vi "REPORT TXT.vi"(6 "Dati collaudo":T1, 8 "template (empty)":path, 9 "BOLLETTINO":string[][](array[string]), 10 "Codice":string, 11 "report file path":path) -> ()   [LabVIEW 2019]
uses:
  <vilib>/Utility/NIReport.llb/NI_report.lvclass
  <vilib>/addons/_office/NI_ReportGenerationToolkit.lvlib
  <vilib>/Utility/NIReport.llb/Excel/NI_Excel.lvclass
  <vilib>/addons/database/NI_Database_API.lvlib
  <vilib>/addons/database/_DB Variant To Data/Database Variant To Data.xnode
  Global percorso impostazioni.vi
  <vilib>/addons/_office/excel.llb/Excel Easy Table (str).vi
  <vilib>/Utility/file.llb/Write Delimited Spreadsheet (string).vi
  TypeDef/Dati collaudo.ctl
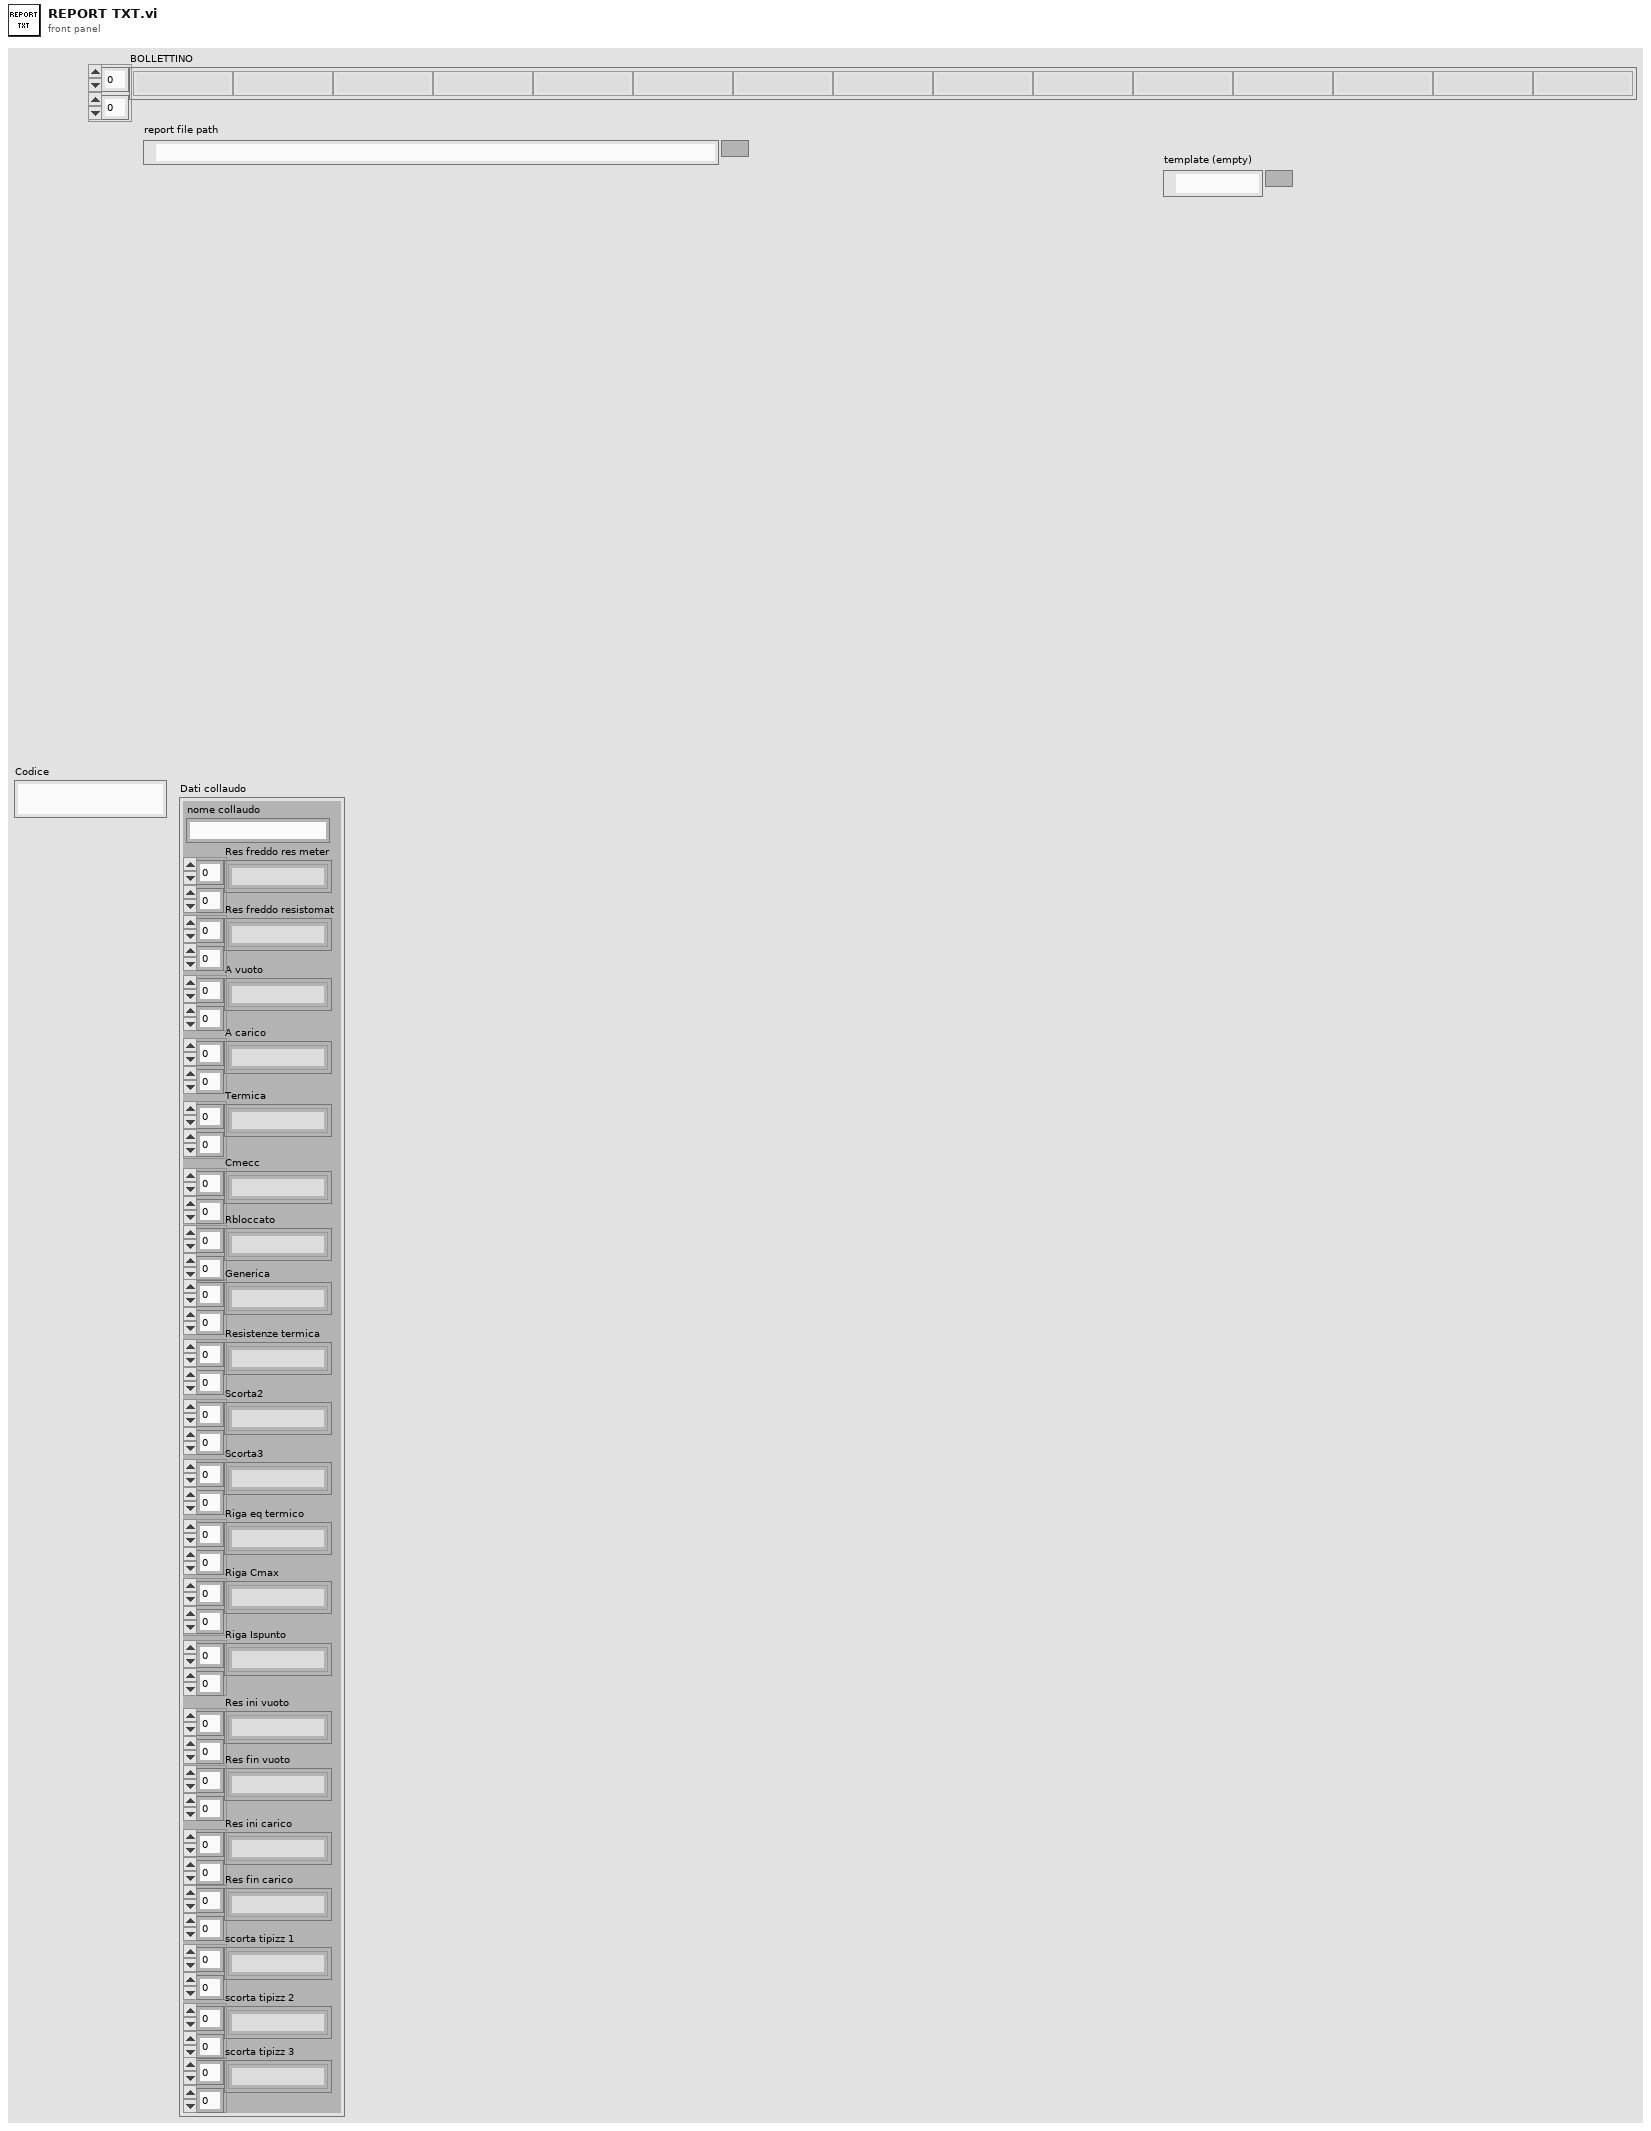
[diagram p1: front panel]
types:
  T1 = typedef "Dati collaudo.ctl" = cluster{"nome collaudo":string, "Res freddo res meter":string[][], "Res freddo resistomat":string[][], "A vuoto":string[][], "A carico":string[][], "Termica":string[][], "Cmecc":string[][], "Rbloccato":string[][], "Generica":string[][], "Resistenze termica":string[][], "Scorta2":string[][], "Scorta3":string[][], "Riga eq termico":string[][], "Riga Cmax":string[][], "Riga Ispunto":string[][], "Res ini vuoto":string[][], "Res fin vuoto":string[][], "Res ini carico":string[][], "Res fin carico":string[][], "scorta tipizz 1":string[][], "scorta tipizz 2":string[][], "scorta tipizz 3":string[][]}
  T2 = cluster{"BANCO":string, "ANNO":string, "PROGRESSIVO":string, "TIPO PROVA":string, "PROVA SPECIALE ?":string, "DATA":string}
  T3 = typedef "NI_Database_API.lvlib/Conn ObjectReference.ctl" = refnum<k1>
  T4 = typedef "Curve prova.ctl" = cluster{"Curva 1":string[][], "Curva 2":string[][], "Curva 3":string[][]}
  T5 = enum16{"maximized", "minimized", "normal", "no change"}
  T6 = enum16{"Standard Report", "HTML", "Word", "Excel"}
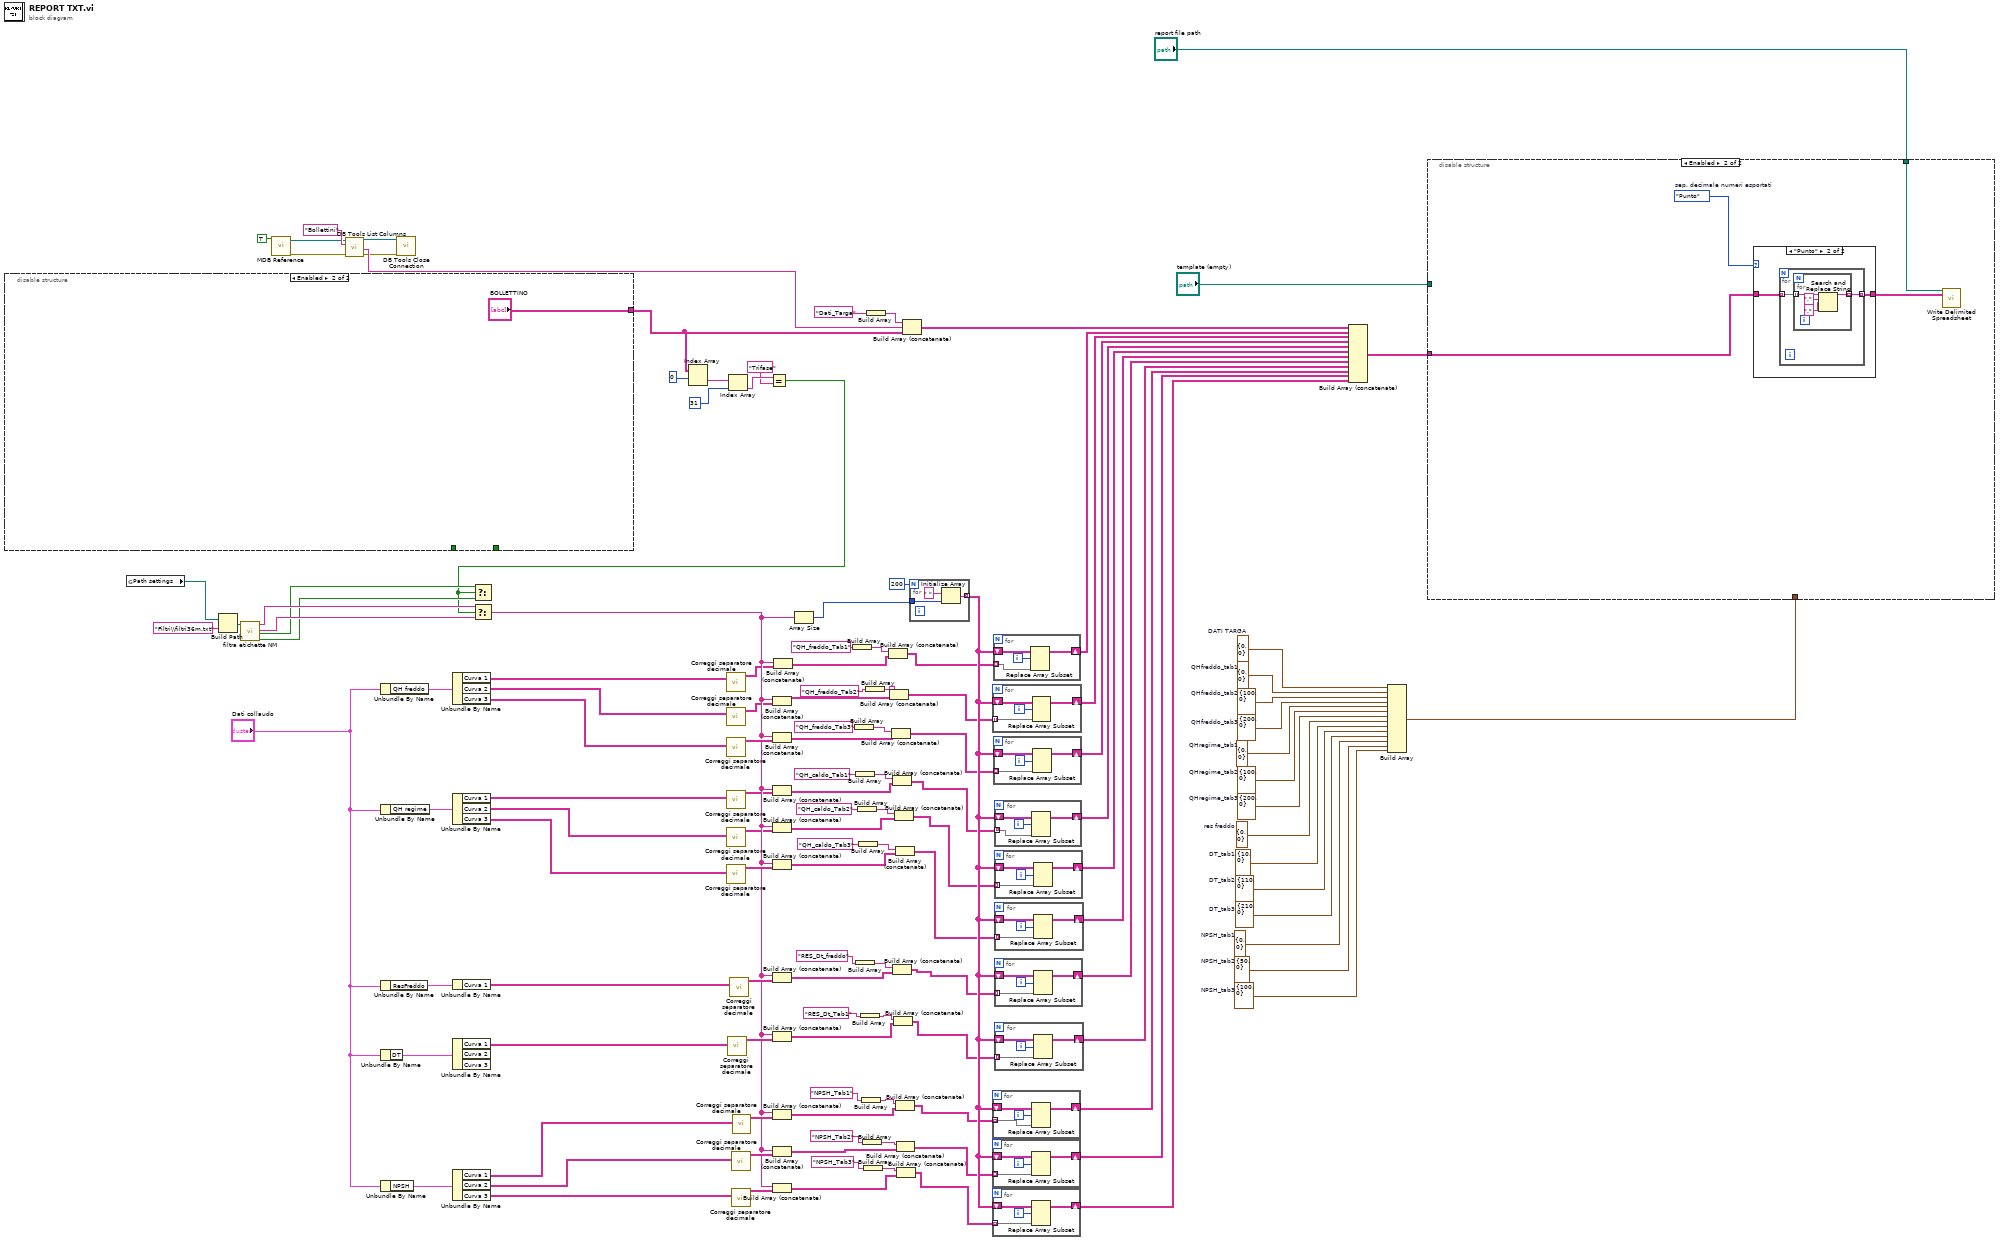
[diagram p0: block diagram]
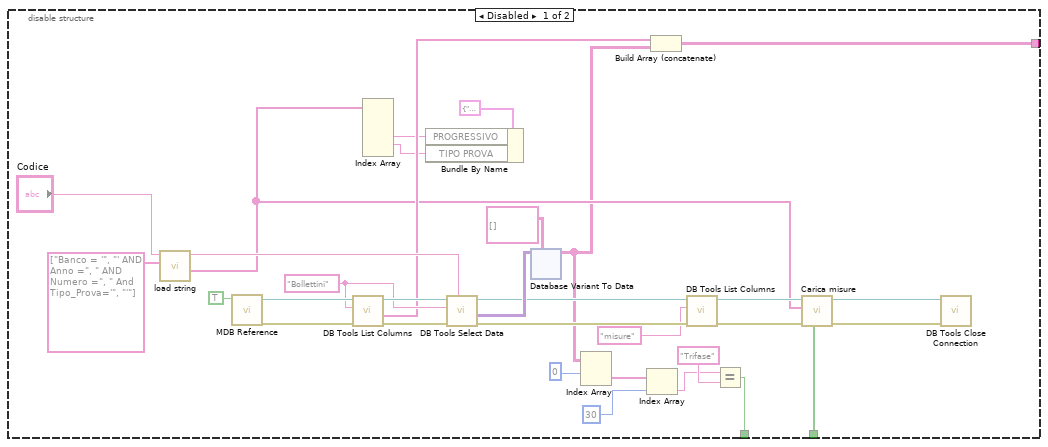
[diagram p2: hidden frame]
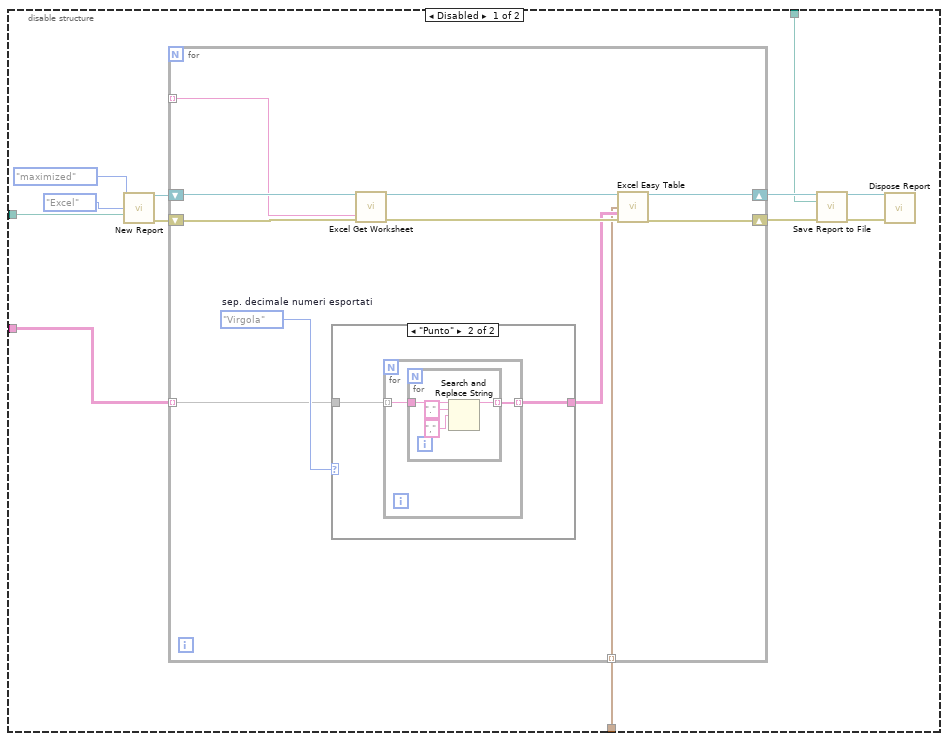
[diagram p3: hidden frame]
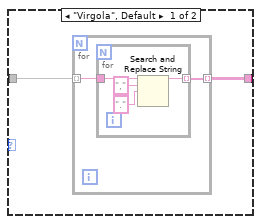
[diagram p4: hidden frame]
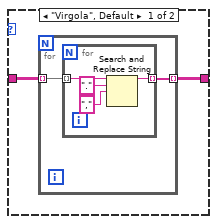
[diagram p5: hidden frame]
diagram:
  w114 = cluster{"row":i32, "column":i32} {"row"=100, "column"=0}  # NPSH_tab3
  w115 = cluster{"row":i32, "column":i32} {"row"=50, "column"=0}  # NPSH_tab2
  w116 = cluster{"row":i32, "column":i32} {"row"=0, "column"=0}  # NPSH_tab1
  w117 = cluster{"row":i32, "column":i32} {"row"=210, "column"=0}  # DT_tab3
  w118 = cluster{"row":i32, "column":i32} {"row"=110, "column"=0}  # DT_tab2
  w119 = cluster{"row":i32, "column":i32} {"row"=10, "column"=0}  # DT_tab1
  w120 = cluster{"row":i32, "column":i32} {"row"=0, "column"=0}  # res freddo
  w121 = cluster{"row":i32, "column":i32} {"row"=200, "column"=0}  # QHregime_tab3
  w122 = cluster{"row":i32, "column":i32} {"row"=100, "column"=0}  # QHregime_tab2
  w123 = cluster{"row":i32, "column":i32} {"row"=0, "column"=0}  # QHregime_tab1
  w124 = cluster{"row":i32, "column":i32} {"row"=200, "column"=0}  # QHfreddo_tab3
  w125 = cluster{"row":i32, "column":i32} {"row"=100, "column"=0}  # QHfreddo_tab2
  w126 = cluster{"row":i32, "column":i32} {"row"=0, "column"=0}  # QHfreddo_tab1
  w127 = cluster{"row":i32, "column":i32} {"row"=0, "column"=0}  # DATI TARGA
  n1 = disable-structure shown="Enabled" {
    disable-tunnel: [w132 _] -> _
    disable-tunnel: _ -> [w131 _]
    disable-tunnel: [w130 "BOLLETTINO"] -> w20
    frame Disabled {
      w152 = "Bollettini" ("table")
      n2 = call "load string.vi"("Array in"=string[] ["Banco = '", "' AND Anno =", " AND Numero =", " And Tipo_Prova='", "'"], "Codice"="Codice") -> ("ID bollettino"=w139:string[], "String command"=w157:string)  [unwired: 7 in, 1 out]
      n3 = call "MDB Reference.vi"("Collaudi T/motori F"=TRUE ("NM?")) -> ("error out"=w154:errorcluster, "Refnum out"=w156:T3)  [unwired: 8 in, 1 out]
      n4 = call <vilib>:"DB Tools List Columns.vi"("error in (no error)"=w154, "table"=w152, "connection reference"=w156) -> ("error out"=w153:errorcluster, "columns"=w151:string[], "connection reference out"=w155:T3)  [unwired: 1 in, 1 out]
      n5 = Index Array(array=w139) -> (element #3=w146:string, element #4=w145:string)  [unwired: 5 in, 3 out]
      n6 = Bundle By Name(cluster=T2 {"BANCO"="0", "ANNO"="17", "PROGRESSIVO"="12", "TIPO PROVA"="F", "PROVA SPECIALE ?"="NO", "DATA"="29/11/2017 10:25:21"} ("bollettino"), "PROGRESSIVO"=w146, "TIPO PROVA"=w145) -> ()  [unwired: 1 out]
      n7 = call <vilib>:"DB Tools Select Data.vi"("condition"=w157, "error in (no error)"=w153, "table"=w152, "connection reference"=w155) -> ("error out"=w150:errorcluster, "data"=w159:variant[][], "connection reference out"=w149:T3)  [unwired: 2 in]
      n8 = xnode "Database Variant To Data"("database variant"=w159, "type"=string[][] [] ("Item Names")) -> ("data"=w133:string[][])  [unwired: 1 in, 1 out]
      n9 = Index Array(array=w133, index (row)=0 ("disabled index (col)")) -> (element=w135:string[])  [unwired: 1 in]
      n10 = Index Array(array=w135, index=30) -> (element=w137:string)
      n11 = Build Array (concatenate)(w151, w133) -> (w130:string[][])
      n12 = call <vilib>:"DB Tools List Columns.vi"("error in (no error)"=w150, "table"="misure", "connection reference"=w149) -> ("error out"=w144:errorcluster, "connection reference out"=w143:T3)  [unwired: 1 in, 2 out]
      n13 = Equal?(x=w137, y="Trifase") -> (x = y?=w132:bool)
      n14 = call "Carica misure.vi"("Filtro 3ph6ch"=w131, "error in (no error)"=w144, "ID bollettino"=w139, "Refnum in"=w143) -> ("error out"=w141:errorcluster, "Refnum out"=w142:T3)  [unwired: 5 in, 1 out]
      n15 = call <vilib>:"DB Tools Close Connection.vi"("error in (no error)"=w141, "connection reference"=w142) -> ()  [unwired: 5 in, 1 out]
    }
    frame Enabled {
    }
  }
  n16 = global read "Global percorso impostazioni.vi" "Path settings"() -> (w1:path)
  n17 = Build Path(base path=w1, name or relative path="Filtri\\filtri36m.txt") -> (appended path=w110:path)
  n18 = call "filtra etichette NM.vi"("File filtri path"=w110) -> ("Array 3ph3ch"=w109:string[], "Array 1ph"=w108:string[], "Filtro 3ph3ch"=w107:bool[], "Filtro 1ph"=w106:bool[])  [unwired: 11 in, 4 out]
  n19 = call "MDB Reference.vi"("Collaudi T/motori F"=TRUE ("NM?")) -> ("error out"=w32:errorcluster, "Refnum out"=w31:T3)  [unwired: 8 in, 1 out]
  n20 = call <vilib>:"DB Tools List Columns.vi"("error in (no error)"=w32, "table"="Bollettini", "connection reference"=w31) -> ("error out"=w27:errorcluster, "columns"=w28:string[], "connection reference out"=w26:T3)  [unwired: 1 in, 1 out]
  n21 = Unbundle By Name("Dati collaudo") -> ("QH freddo"=w101:T4)
  n22 = Unbundle By Name("Dati collaudo") -> ("QH regime"=w102:T4)
  n23 = Unbundle By Name("Dati collaudo") -> ("ResFreddo"=w104:cluster{"Curva 1":string[][]})
  n24 = Unbundle By Name("Dati collaudo") -> ("DT"=w103:T4)
  n25 = Unbundle By Name("Dati collaudo") -> ("NPSH"=w105:T4)
  n26 = call <vilib>:"DB Tools Close Connection.vi"("error in (no error)"=w27, "connection reference"=w26) -> ()  [unwired: 5 in, 1 out]
  n27 = Unbundle By Name(w101) -> ("Curva 1"=w10:string[][], "Curva 2"=w8:string[][], "Curva 3"=w16:string[][])
  n28 = Unbundle By Name(w102) -> ("Curva 1"=w12:string[][], "Curva 2"=w14:string[][], "Curva 3"=w15:string[][])
  n29 = Unbundle By Name(w104) -> ("Curva 1"=w6:string[][])
  n30 = Unbundle By Name(w103) -> ("Curva 1"=w5:string[][])  [unwired: 2 out]
  n31 = Unbundle By Name(w105) -> ("Curva 1"=w4:string[][], "Curva 2"=w3:string[][], "Curva 3"=w2:string[][])
  n32 = Index Array(array=w20, index (row)=0 ("disabled index (col)")) -> (element=w24:string[])  [unwired: 1 in]
  n33 = call "Correggi separatore decimale.vi"("Array in"=w10) -> ("Array out"=w9:string[][])  [unwired: 10 in]
  n34 = call "Correggi separatore decimale.vi"("Array in"=w8) -> ("Array out"=w7:string[][])  [unwired: 10 in]
  n35 = call "Correggi separatore decimale.vi"("Array in"=w16) -> ("Array out"=w99:string[][])  [unwired: 10 in]
  n36 = call "Correggi separatore decimale.vi"("Array in"=w12) -> ("Array out"=w11:string[][])  [unwired: 10 in]
  n37 = call "Correggi separatore decimale.vi"("Array in"=w14) -> ("Array out"=w13:string[][])  [unwired: 10 in]
  n38 = call "Correggi separatore decimale.vi"("Array in"=w15) -> ("Array out"=w98:string[][])  [unwired: 10 in]
  n39 = call "Correggi separatore decimale.vi"("Array in"=w5) -> ("Array out"=w96:string[][])  [unwired: 10 in]
  n40 = Index Array(array=w24, index=31) -> (element=w22:string)
  n41 = call "Correggi separatore decimale.vi"("Array in"=w6) -> ("Array out"=w97:string[][])  [unwired: 10 in]
  n42 = call "Correggi separatore decimale.vi"("Array in"=w3) -> ("Array out"=w94:string[][])  [unwired: 10 in]
  n43 = call "Correggi separatore decimale.vi"("Array in"=w2) -> ("Array out"=w95:string[][])  [unwired: 10 in]
  n44 = call "Correggi separatore decimale.vi"("Array in"=w4) -> ("Array out"=w93:string[][])  [unwired: 10 in]
  n45 = Equal?(x=w22, y="Trifase") -> (x = y?=w19:bool)
  n46 = Select(t=w107, s=w19, f=w106) -> ()  [unwired: 1 out]
  n47 = Select(t=w109, s=w19, f=w108) -> (s? t:f=w17:string[])
  n48 = Build Array (concatenate)(w17, w7) -> (w73:string[][])
  n49 = Build Array (concatenate)(w17, w99) -> (w67:string[][])
  n50 = Build Array (concatenate)(w17, w11) -> (w64:string[][])
  n51 = Build Array (concatenate)(w17, w13) -> (w57:string[][])
  n52 = Build Array (concatenate)(w17, w98) -> (w55:string[][])
  n53 = Build Array (concatenate)(w17, w97) -> (w52:string[][])
  n54 = Build Array (concatenate)(w17, w96) -> (w49:string[][])
  n55 = Build Array (concatenate)(w17, w93) -> (w44:string[][])
  n56 = Build Array (concatenate)(w17, w94) -> (w39:string[][])
  n57 = Build Array (concatenate)(w17, w95) -> (w35:string[][])
  n58 = Build Array (concatenate)(w17, w9) -> (w75:string[][])
  n59 = Array Size(array=w17) -> (size(s)=w18:i32)
  n60 = Build Array("QH_freddo_Tab1") -> (w77:string[])
  n61 = Build Array("QH_freddo_Tab3") -> (w68:string[])
  n62 = Build Array("QH_caldo_Tab1") -> (w65:string[])
  n63 = Build Array("RES_Dt_freddo") -> (w53:string[])
  n64 = Build Array("QH_caldo_Tab2") -> (w60:string[])
  n65 = Build Array("QH_caldo_Tab3") -> (w59:string[])
  n66 = Build Array("RES_Dt_Tab1") -> (w46:string[])
  n67 = Build Array("NPSH_Tab1") -> (w45:string[])
  n68 = Build Array("NPSH_Tab2") -> (w40:string[])
  n69 = Build Array("NPSH_Tab3") -> (w37:string[])
  n70 = Build Array("QH_freddo_Tab2") -> (w71:string[])
  n71 = Build Array("Dati_Targa") -> (w29:string[])
  n72 = Build Array (concatenate)(w77, w75) -> (w74:string[][])
  n73 = Build Array (concatenate)(w71, w73) -> (w72:string[][])
  n74 = Build Array (concatenate)(w68, w67) -> (w66:string[][])
  n75 = Build Array (concatenate)(w65, w64) -> (w63:string[][])
  n76 = Build Array (concatenate)(w53, w52) -> (w51:string[][])
  n77 = Build Array (concatenate)(w46, w49) -> (w48:string[][])
  n78 = Build Array (concatenate)(w60, w57) -> (w56:string[][])
  n79 = Build Array (concatenate)(w59, w55) -> (w54:string[][])
  n80 = Build Array (concatenate)(w45, w44) -> (w43:string[][])
  n81 = Build Array (concatenate)(w40, w39) -> (w38:string[][])
  n82 = Build Array (concatenate)(w37, w35) -> (w34:string[][])
  n83 = Build Array (concatenate)(w29, w28, w20) -> (w82:string[][])
  n84 = for {
    N: 200 -> [_]
    tunnel: w18 -> [w208]
    tunnel: [w207] -> w80 mode=indexing
    n85 = Initialize Array(" ", w208) -> (w207:string[])
  }
  n86 = for {
    shift-right: [w211] -> w85
    shift-left: w80 -> [w213]
    tunnel: w43 -> [w210] mode=indexing
    i -> [w212]
    n87 = Replace Array Subset(array=w213, new element=w210, index (row)=w212) -> (w211:string[][])  [unwired: 1 in]
  }
  n88 = for {
    shift-right: [w215] -> w84
    shift-left: w80 -> [w217]
    tunnel: w38 -> [w214] mode=indexing
    i -> [w216]
    n89 = Replace Array Subset(array=w217, new element=w214, index (row)=w216) -> (w215:string[][])  [unwired: 1 in]
  }
  n90 = for {
    shift-right: [w219] -> w83
    shift-left: w80 -> [w221]
    tunnel: w34 -> [w218] mode=indexing
    i -> [w220]
    n91 = Replace Array Subset(array=w221, new element=w218, index (row)=w220) -> (w219:string[][])  [unwired: 1 in]
  }
  n92 = for {
    shift-right: [w223] -> w90
    shift-left: w80 -> [w225]
    tunnel: w72 -> [w222] mode=indexing
    i -> [w224]
    n93 = Replace Array Subset(array=w225, new element=w222, index (row)=w224) -> (w223:string[][])  [unwired: 1 in]
  }
  n94 = for {
    tunnel: w74 -> [w228] mode=indexing
    shift-right: [w226] -> w91
    shift-left: w80 -> [w229]
    i -> [w227]
    n95 = Replace Array Subset(array=w229, new element=w228, index (row)=w227) -> (w226:string[][])  [unwired: 1 in]
  }
  n96 = for {
    shift-right: [w231] -> w89
    shift-left: w80 -> [w233]
    tunnel: w66 -> [w230] mode=indexing
    i -> [w232]
    n97 = Replace Array Subset(array=w233, new element=w230, index (row)=w232) -> (w231:string[][])  [unwired: 1 in]
  }
  n98 = for {
    shift-right: [w235] -> w87
    shift-left: w80 -> [w237]
    tunnel: w56 -> [w234] mode=indexing
    i -> [w236]
    n99 = Replace Array Subset(array=w237, new element=w234, index (row)=w236) -> (w235:string[][])  [unwired: 1 in]
  }
  n100 = for {
    shift-right: [w239] -> w78
    shift-left: w80 -> [w241]
    tunnel: w51 -> [w238] mode=indexing
    i -> [w240]
    n101 = Replace Array Subset(array=w241, new element=w238, index (row)=w240) -> (w239:string[][])  [unwired: 1 in]
  }
  n102 = for {
    tunnel: w63 -> [w244] mode=indexing
    shift-right: [w242] -> w88
    shift-left: w80 -> [w245]
    i -> [w243]
    n103 = Replace Array Subset(array=w245, new element=w244, index (row)=w243) -> (w242:string[][])  [unwired: 1 in]
  }
  n104 = for {
    shift-right: [w247] -> w86
    shift-left: w80 -> [w249]
    tunnel: w54 -> [w246] mode=indexing
    i -> [w248]
    n105 = Replace Array Subset(array=w249, new element=w246, index (row)=w248) -> (w247:string[][])  [unwired: 1 in]
  }
  n106 = for {
    shift-right: [w251] -> w79
    shift-left: w80 -> [w253]
    tunnel: w48 -> [w250] mode=indexing
    i -> [w252]
    n107 = Replace Array Subset(array=w253, new element=w250, index (row)=w252) -> (w251:string[][])  [unwired: 1 in]
  }
  n108 = Build Array (concatenate)(w82, w91, w90, w89, w88, w87, w86, w78, w79, w85, w84, w83) -> (w128:string[][])
  n109 = Build Array(w127, w126, w125, w124, w123, w122, w121, w120, w119, w118, w117, w116, w115, w114) -> (w113:cluster{"row":i32, "column":i32}[])
  n110 = disable-structure shown="Enabled" {
    disable-tunnel: "template (empty)" -> [w266 _]
    disable-tunnel: w128 -> [w261 w294]
    disable-tunnel: w113 -> [w259 _]
    disable-tunnel: "report file path" -> [w254 w297]
    frame Disabled {
      n111 = call <vilib>:"New Report.vi"("window state (normal)"=T5."maximized", "report type"=T6."Excel", "template (empty)"=w266) -> ("report out"=w264:refnum<class "NI_report.lvclass">, "error out"=w262:errorcluster)  [unwired: 11 in]
      n112 = for {
        shift-right: [w277] -> w256
        shift-left: w264 -> [w276]
        tunnel: [w274] -> w263 mode=indexing
        shift-right: [w271] -> w258
        shift-left: w262 -> [w273]
        tunnel: w261 -> [w269] mode=indexing
        tunnel: w259 -> [w267] mode=indexing
        w270 = enum16{"Virgola", "Punto"}."Virgola"  # sep. decimale numeri esportati
        n113 = case shown="\"Punto\"" w270 {
          tunnel: w269 -> [w279 w287]
          tunnel: [w278 w286] -> w268
          frame "Virgola", Default {
            n114 = for {
              tunnel: w279 -> [w281] mode=indexing
              tunnel: [w280] -> w278 mode=indexing
              n115 = for {
                tunnel: w281 -> [w285]
                tunnel: [w282] -> w280 mode=indexing
                n116 = Search and Replace String(input string=w285, search string=",", replace string="." ("search string")) -> (result string=w282:string)  [unwired: 5 in, 3 out]
              }
            }
          }
          frame "Punto" {
            n117 = for {
              tunnel: w287 -> [w289] mode=indexing
              tunnel: [w288] -> w286 mode=indexing
              n118 = for {
                tunnel: w289 -> [w293]
                tunnel: [w290] -> w288 mode=indexing
                n119 = Search and Replace String(input string=w293, search string=".", replace string="," ("search string")) -> (result string=w290:string)  [unwired: 5 in, 3 out]
              }
            }
          }
        }
        n120 = call <vilib>:"Excel Get Worksheet.vi"("report in"=w276, "error in (no error)"=w273, "name (\"\")"=w274) -> ("report out"=w275:refnum<class "NI_report.lvclass">, "error out"=w272:errorcluster)  [unwired: 11 in]
        n121 = call-poly <vilib>:"Excel Easy Table.vi"("report in"=w275, "start (0, 0)"=w267, "text data"=w268, "error in (no error)"=w272) -> ("report out"=w277:refnum<class "NI_report.lvclass">, "error out"=w271:errorcluster)  [unwired: 7 in, 3 out]
      }
      n122 = call-dynamic "Save Report to File.vi"("report in"=w256, "report file path"=w254, "error in (no error)"=w258) -> ("report out"=w255:refnum<class "NI_report.lvclass">, "error out"=w257:errorcluster)  [unwired: 11 in]
      n123 = call-dynamic "Dispose Report.vi"("report in"=w255, "error in (no error)"=w257) -> ()  [unwired: 13 in, 1 out]
    }
    frame Enabled {
      w296 = enum16{"Virgola", "Punto"}."Punto"  # sep. decimale numeri esportati
      n124 = case shown="\"Punto\"" w296 {
        tunnel: w294 -> [w299 w307]
        tunnel: [w298 w306] -> w295
        frame "Virgola", Default {
          n125 = for {
            tunnel: w299 -> [w301] mode=indexing
            tunnel: [w300] -> w298 mode=indexing
            n126 = for {
              tunnel: w301 -> [w305] mode=indexing
              tunnel: [w302] -> w300 mode=indexing
              n127 = Search and Replace String(input string=w305, search string=".", replace string="," ("search string")) -> (result string=w302:string)  [unwired: 5 in, 3 out]
            }
          }
        }
        frame "Punto" {
          n128 = for {
            tunnel: w307 -> [w309] mode=indexing
            tunnel: [w308] -> w306 mode=indexing
            n129 = for {
              tunnel: w309 -> [w313] mode=indexing
              tunnel: [w310] -> w308 mode=indexing
              n130 = Search and Replace String(input string=w313, search string=",", replace string="." ("search string")) -> (result string=w310:string)  [unwired: 5 in, 3 out]
            }
          }
        }
      }
      n131 = call-poly <vilib>:"Write Delimited Spreadsheet.vi"("file path (dialog if empty)"=w297, "2D data"=w295) -> ()  [unwired: 12 in, 2 out]
    }
  }
